vi "LoadUI.vi"(8 "error in (no error)":errorcluster, 10 "Actor In":refnum<class "Actor.lvclass">, 11 "Analyser in":refnum<class "Analyser.lvclass">) -> (0 "error out":errorcluster, 3 "Analyser out":refnum<class "Analyser.lvclass">)   [LabVIEW 2020, in "Analyser.lvlib" / "Analyser.lvclass"]
uses:
  Analyser.lvclass
  C:/Program Files/National Instruments/LabVIEW 2020/vi.lib/ActorFramework/Actor/Actor.lvclass
  <vilib>/ActorFramework/Actor/Actor.lvclass
  Analyser.lvclass/Analyser.ctl
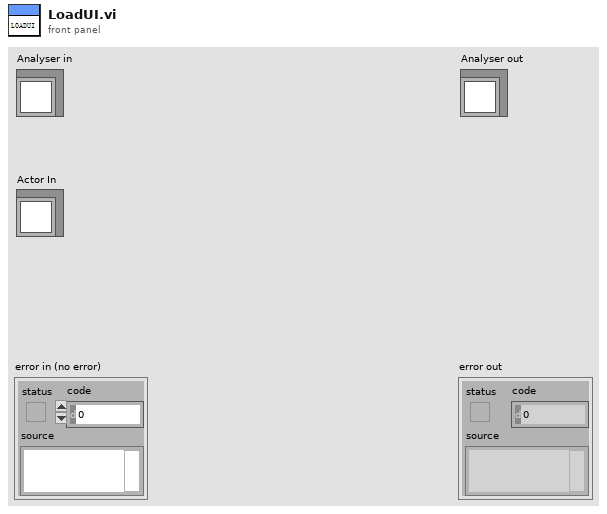
[diagram p1: front panel]
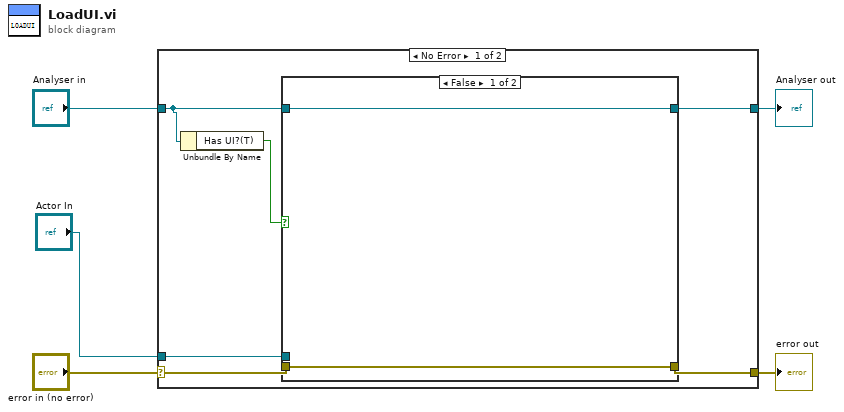
[diagram p0: block diagram]
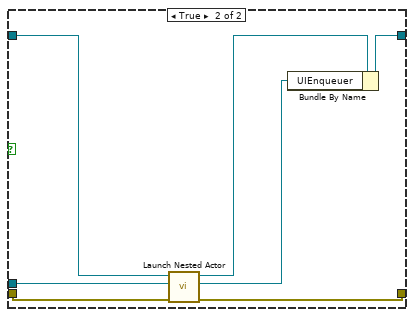
[diagram p2: hidden frame]
diagram:
  n1 = case shown="No Error" "error in (no error)" {
    selector: "error in (no error)" -> [w11 w22]
    tunnel: [w10 w22] -> w4
    tunnel: [w8 w21] -> w2
    tunnel: "Analyser in" -> [w7 w21]
    tunnel: "Actor In" -> [w9 _]
    frame No Error {
      n2 = Unbundle By Name(w7) -> ("Has UI?(T)"=w6:bool)
      n3 = case shown="False" w6 {
        tunnel: w11 -> [w12 w20]
        tunnel: [w12 w19] -> w10
        tunnel: w7 -> [w13 w18]
        tunnel: w9 -> [_ w16]
        tunnel: [w13 w15] -> w8
        frame False {
        }
        frame True {
          n4 = call <vilib>:"Launch Nested Actor.vi"("error in (no error)"=w20, "Nested Actor"=w16, "Caller Actor in"=w18) -> ("error out"=w19:errorcluster, "Nested Actor's Enqueuer"=w14:refnum<class "Message Enqueuer.lvclass">, "Caller Actor out"=w17:refnum<class "Analyser.lvclass">)  [unwired: 6 in]
          n5 = Bundle By Name(cluster=w17, "UIEnqueuer"=w14) -> (w15:refnum<class "Analyser.lvclass">)
        }
      }
    }
    frame Error {
    }
  }
  "error out" <- w4
  "Analyser out" <- w2
